vi "New AbstractBuilder.vi"(0 "reference in":refnum<class "AbstractBuilder.lvclass">, 5 "error in (no error)":errorcluster) -> (14 "reference out":refnum<class "AbstractBuilder.lvclass">, 19 "error out":errorcluster)   [LabVIEW 2015, in "AbstractBuilder.lvclass"]
uses:
  AbstractBuilder.lvclass
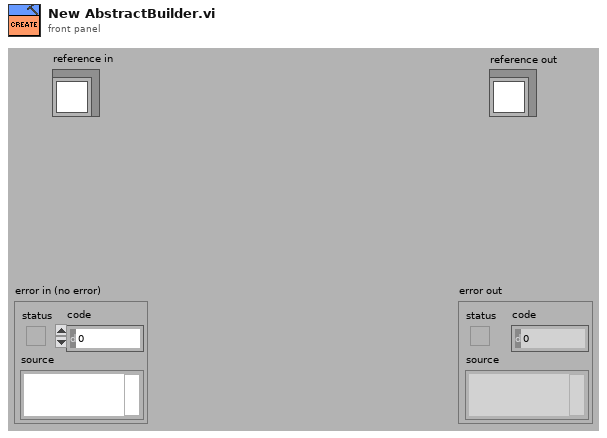
[diagram p1: front panel]
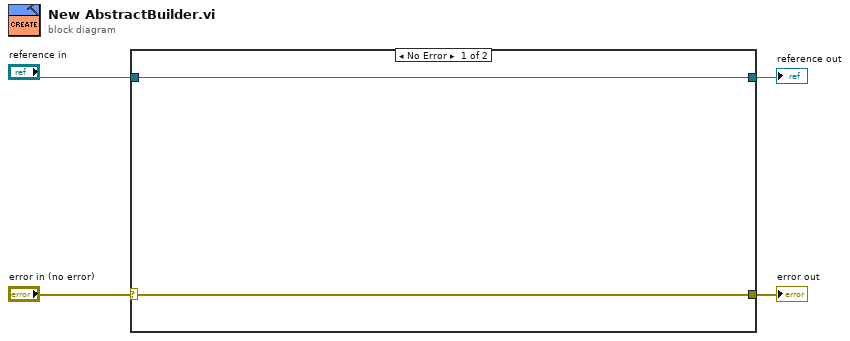
[diagram p0: block diagram]
diagram:
  n1 = case shown="No Error" "error in (no error)" {
    selector: "error in (no error)" -> [w5 w8]
    tunnel: [w5 w8] -> w3
    tunnel: "reference in" -> [w6 w7]
    tunnel: [w6 w7] -> w1
    frame No Error {
    }
    frame Error {
    }
  }
  "error out" <- w3
  "reference out" <- w1
